vi "矩阵加边框.vi"(4 "下边框宽度":i32, 5 "复制面阵边缘作为边框值":bool, 6 "上边框宽度":i32, 8 "右边框宽度":i32, 9 "左边框宽度":i32, 10 "边框值":dbl, 11 "原面阵":dbl[][](array[numeric])) -> (3 "加边框面阵":dbl[][](array[numeric]))   [LabVIEW 2016]
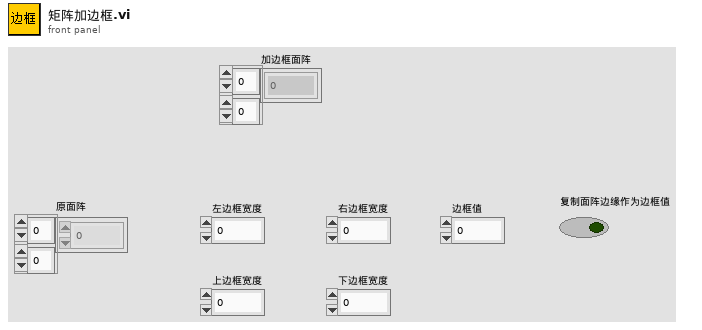
[diagram p1: front panel]
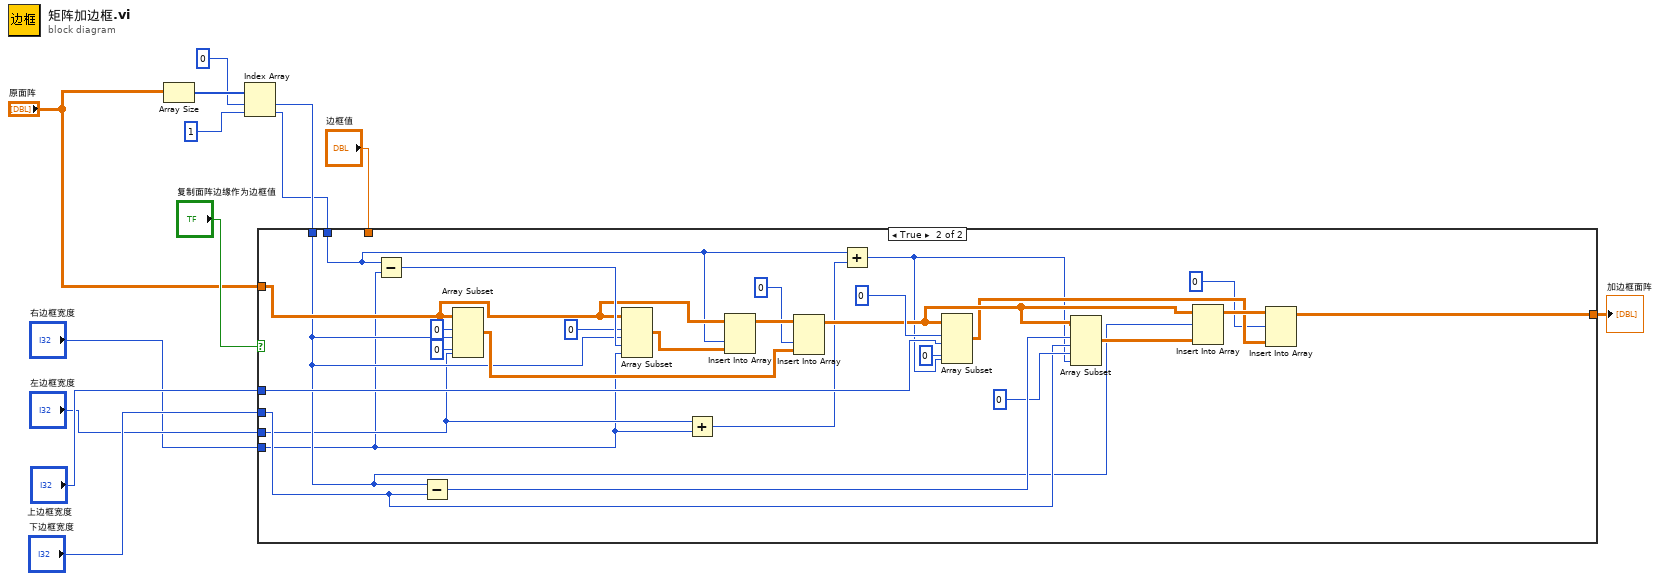
[diagram p0: block diagram]
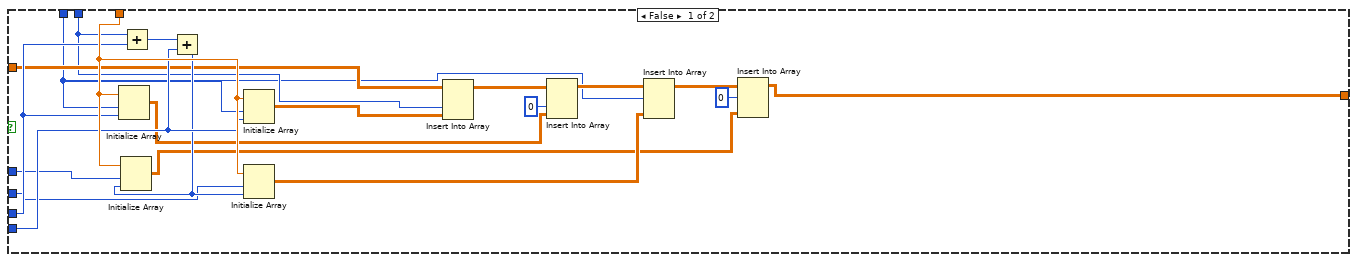
[diagram p2: hidden frame]
diagram:
  n1 = Array Size(array="原面阵") -> (size(s)=w13:i32[])
  n2 = Index Array(array=w13, index #1=0 ("index"), index #2=1 ("index")) -> (element #1=w8:i32, element #2=w7:i32)
  n3 = case shown="True" "复制面阵边缘作为边框值" {
    tunnel: "边框值" -> [w33 _]
    tunnel: w8 -> [w17 w42]
    tunnel: w7 -> [w21 w45]
    tunnel: "上边框宽度" -> [w28 w49]
    tunnel: "下边框宽度" -> [w27 w46]
    tunnel: "左边框宽度" -> [w31 w37]
    tunnel: "右边框宽度" -> [w30 w36]
    tunnel: "原面阵" -> [w25 w56]
    tunnel: [w14 w38] -> w1
    frame False {
      n4 = Initialize Array(w33, w17, w31) -> (w20:dbl[][])
      n5 = Add(x=w21, y=w31) -> (x+y=w32:i32)
      n6 = Add(x=w32, y=w30) -> (x+y=w29:i32)
      n7 = Initialize Array(w33, w28, w29) -> (w16:dbl[][])
      n8 = Initialize Array(w33, w17, w30) -> (w26:dbl[][])
      n9 = Initialize Array(w33, w27, w29) -> (w18:dbl[][])
      n10 = Insert Into Array(array=w25, index (col)=w21, new element=w26) -> (w24:dbl[][])  [unwired: 1 in]
      n11 = Insert Into Array(array=w24, index (col)=0 ("disabled index (col)"), new element=w20) -> (w23:dbl[][])  [unwired: 1 in]
      n12 = Insert Into Array(array=w23, index (row)=w17, new element=w18) -> (w22:dbl[][])  [unwired: 1 in]
      n13 = Insert Into Array(array=w22, index (row)=0, new element=w16) -> (w14:dbl[][])  [unwired: 1 in]
    }
    frame True {
      n14 = Subtract(x=w45, y=w36) -> (x-y=w58:i32)
      n15 = Subtract(x=w42, y=w46) -> (x-y=w48:i32)
      n16 = Array Subset(array=w56, index (row)=0 ("index"), length (row)=w42, index (col)=0 ("index"), length (col)=w37) -> (w53:dbl[][])
      n17 = Array Subset(array=w56, index (row)=0 ("index"), length (row)=w42, index (col)=w58, length (col)=w36) -> (w55:dbl[][])
      n18 = Add(x=w37, y=w36) -> (x+y=w34:i32)
      n19 = Insert Into Array(array=w56, index (col)=w45, new element=w55) -> (w54:dbl[][])  [unwired: 1 in]
      n20 = Insert Into Array(array=w54, index (col)=0 ("disabled index (col)"), new element=w53) -> (w44:dbl[][])  [unwired: 1 in]
      n21 = Add(x=w45, y=w34) -> (x+y=w35:i32)
      n22 = Array Subset(array=w44, index (row)=0 ("index"), length (row)=w49, index (col)=0 ("index"), length (col)=w35) -> (w40:dbl[][])
      n23 = Array Subset(array=w44, index (row)=w48, length (row)=w46, index (col)=0 ("index"), length (col)=w35) -> (w43:dbl[][])
      n24 = Insert Into Array(array=w44, index (row)=w42, new element=w43) -> (w41:dbl[][])  [unwired: 1 in]
      n25 = Insert Into Array(array=w41, index (row)=0, new element=w40) -> (w38:dbl[][])  [unwired: 1 in]
    }
  }
  "加边框面阵" <- w1
